vi "File IO.vi"(8 "error in":errorcluster, 9 "This Scan #":u32, 11 "File IO in":refnum<class "File IO.lvclass">) -> (0 "error out":errorcluster, 3 "File IO out":refnum<class "File IO.lvclass">)   [LabVIEW 2009, in "File IO.lvclass"]
uses:
  File IO.lvclass
  File IO.lvclass/File IO.ctl
  Global/File Locations.vi
panel:
  out "Temp File Path":path
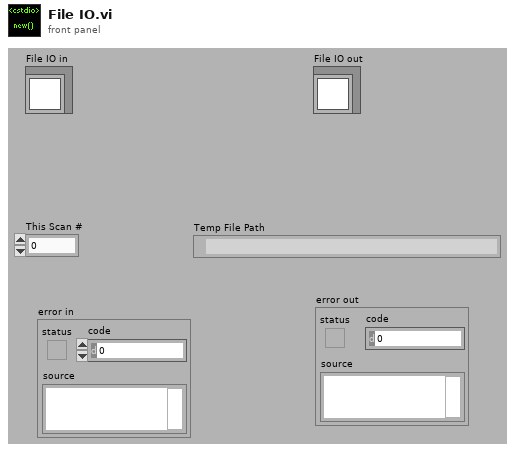
[diagram p1: front panel]
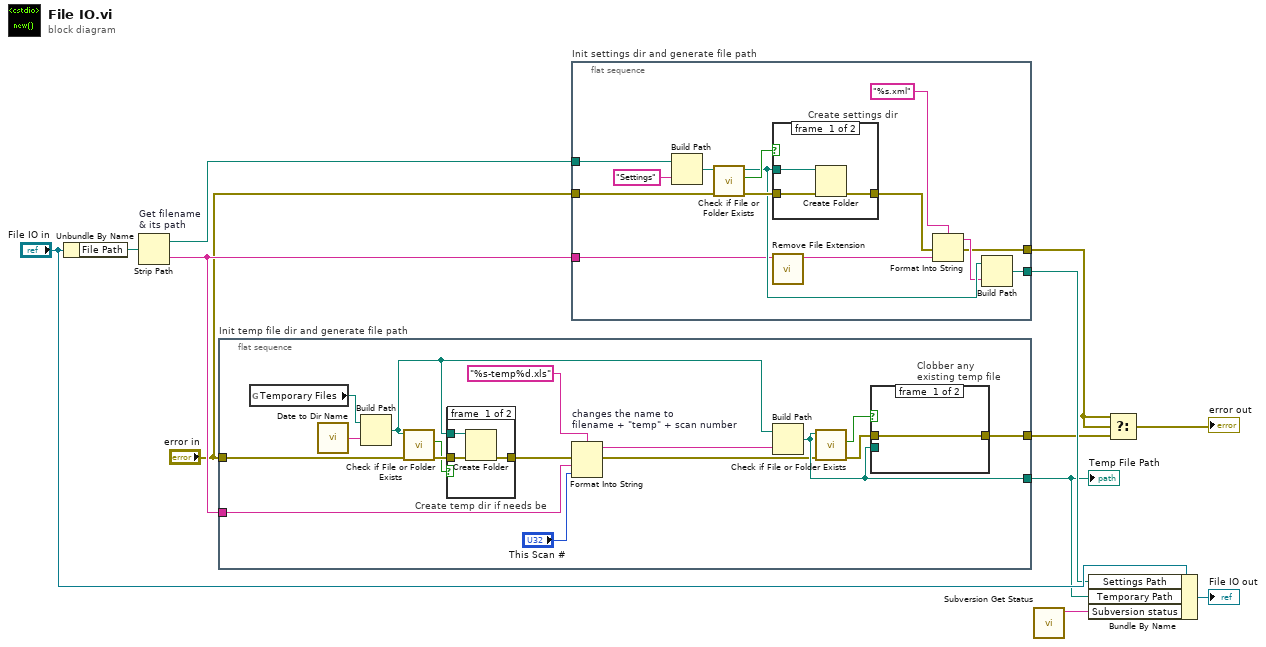
[diagram p0: block diagram]
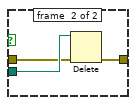
[diagram p3: hidden frame]
diagram:
  n1 = Unbundle By Name("File IO in") -> ("File Path"=w12:path)
  n2 = Strip Path "Get filename\n& its path"(path=w12) -> (stripped path=w9:path, name=w8:string)
  n3 = flat-sequence "Init temp file dir and generate file path" {
    tunnel: [w22] -> w5
    tunnel: [w21] -> w4
    tunnel: w8 -> [w16]
    tunnel: "error in" -> [w13]
    frame #0 {
      n4 = global read "File Locations.vi" "Temporary Files"() -> (w26:path)
      n5 = call "Date to Dir Name.vi"() -> ("Dir Name"=w25:string)
      n6 = Build Path(base path=w26, name or relative path=w25) -> (appended path=w17:path)
      n7 = call <vilib>:"Check if File or Folder Exists.vi"("error in (no error)"=w13, "path"=w17) -> ("error out"=w20:errorcluster, "file or folder exists?"=w18:bool)  [unwired: 8 out]
      n8 = case "Create temp dir if needs be" shown="False" w18 {
        tunnel: w20 -> [w31 w32]
        tunnel: w17 -> [w30 _]
        tunnel: [w29 w32] -> w15
        frame #0 {
          n9 = Create Folder(path (use dialog)=w30, error in=w31) -> (error out=w29:errorcluster)  [unwired: 3 out]
        }
        frame #1 {
        }
      }
      n10 = Format Into String "changes the name to \nfilename + \"temp\" + scan number"(format string="%s-temp%d.xls", error in=w15, w16, "This Scan #") -> (resulting string=w24:string, error out=w14:errorcluster)  [unwired: 1 in]
      n11 = Build Path(base path=w17, name or relative path=w24) -> (appended path=w22:path)
      n12 = call <vilib>:"Check if File or Folder Exists.vi"("error in (no error)"=w14, "path"=w22) -> ("error out"=w19:errorcluster, "file or folder exists?"=w23:bool)  [unwired: 8 out]
      n13 = case "Clobber any\nexisting temp file" shown="True" w23 {
        tunnel: w22 -> [_ w36]
        tunnel: w19 -> [w33 w35]
        tunnel: [w33 w34] -> w21
        frame #0 {
        }
        frame #1 {
          n14 = Delete(path (use dialog)=w36, error in=w35) -> (error out=w34:errorcluster)  [unwired: 5 out]
        }
      }
    }
  }
  n15 = flat-sequence "Init settings dir and generate file path" {
    tunnel: w9 -> [w50]
    tunnel: w8 -> [w44]
    tunnel: [w40] -> w7
    tunnel: "error in" -> [w38]
    tunnel: [w37] -> w3
    frame #0 {
      n16 = Build Path(base path=w50, name or relative path="Settings") -> (appended path=w48:path)
      n17 = call <vilib>:"Check if File or Folder Exists.vi"("error in (no error)"=w38, "path"=w48) -> ("error out"=w46:errorcluster, "file or folder exists?"=w47:bool, "dup path"=w45:path)  [unwired: 7 out]
      n18 = case "Create settings dir" shown="False" w47 {
        tunnel: w46 -> [w53 w54]
        tunnel: [w52 w54] -> w39
        tunnel: w45 -> [w51 _]
        frame #0 {
          n19 = Create Folder(path (use dialog)=w51, error in=w53) -> (error out=w52:errorcluster)  [unwired: 3 out]
        }
        frame #1 {
        }
      }
      n20 = call "Remove File Extension.vi"("filename"=w44) -> ("adjustedfilename"=w42:string)  [unwired: 6 out]
      n21 = Format Into String(format string="%s.xml", error in=w39, w42) -> (resulting string=w41:string, error out=w37:errorcluster)  [unwired: 1 in]
      n22 = Build Path(base path=w45, name or relative path=w41) -> (appended path=w40:path)
    }
  }
  n23 = call "Subversion Get Status.vi"() -> ("SVN Status"=w1:string)  [unwired: 11 out]
  n24 = Bundle By Name(cluster="File IO in", "Settings Path"=w7, "Temporary Path"=w5, "Subversion status"=w1) -> (→"File IO out":refnum<class "File IO.lvclass">)
  n25 = Select(t=w3, s=w3, f=w4) -> (s? t:f=→"error out":errorcluster)
  "Temp File Path" <- w5
